vi "Begin.vi"(8 "error in":errorcluster) -> (0 "error out":T1)   [LabVIEW 2014]
doc: "Called before other user functions, this VI is expected to open initial I/O refnums, load in file data, and do all program initialization. Notice that the <B>error out</B> terminal is simply used for data flow. Wiring it to other structures or subVIs ensures that this VI runs first."
uses:
  ErrorOut.ctl
  <vilib>/Rock Robotics/WPI/SafetyOutput/WPI_SafetyOutputConfigMenu.ctl
  <vilib>/Rock Robotics/WPI/DriverStation/WPI_DriverStationRobotMode2.ctl
  <vilib>/Rock Robotics/WPI/Joystick/WPI_JoystickDeviceEnum.ctl
  <vilib>/Rock Robotics/SystemInterfaces/AI/FPGA_AIGyroChannel.ctl
  Robot Global Data.vi
  <vilib>/Rock Robotics/Network Tables/SD Write String Array.vi
  <vilib>/Rock Robotics/WPI/RobotDrive/WPI_RobotDriveOpen4MotorWithCANTalonSRX.vi
  <vilib>/Rock Robotics/WPI/MotorControl/WPI_MotorControlOpenCANTalonSRX.vi
  <vilib>/Rock Robotics/WPI/Compressor/WPI_CompressorGetSetRefNum.vi
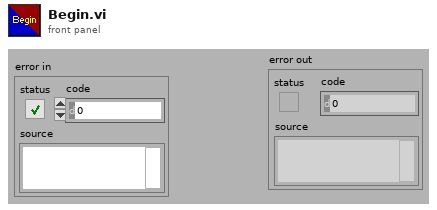
[diagram p1: front panel]
types:
  T1 = typedef "ErrorOut.ctl" = errorcluster
  T2 = typedef "FPGA_AIGyroChannel.ctl" = enum8{"AI 0", "AI 1", "Invalid"}
  T3 = typedef "WPI_JoystickDeviceEnum.ctl" = enum16{"USB 0", "USB 1", "USB 2", "USB 3", "USB 4", "USB 5"}
  T4 = typedef "WPI_DriverStationRobotMode2.ctl" = enum16{"Autonomous Disabled", "Autonomous Enabled", "Teleop Disabled", "Teleop Enabled", "Disconnected", "Finish", "Test Disabled", "Test Enabled", "Emergency Stopped"}
  T5 = typedef "WPI_SafetyOutputConfigMenu.ctl" = enum16{"Enable", "Disable"}
  T6 = typedef "WPI_JoystickDevRef.ctl" = cluster{"Device":T3}
  T7 = typedef "WPI_RobotDriveDevRef.ctl" = cluster{"DevStatus":errorcluster, "Motors[]":T8[], "Square Inputs":bool, "Max Output":dbl}
  T8 = typedef "WPI_MotorControlDeviceRef.ctl" = cluster{"DeviceStatus":errorcluster, "Type":T9, "PWM":cluster{"Controller":T10, "PWM Channel":T11, "DeadBand":T12}, "CAN":cluster{"Device Number":u8, "Control Mode":T13, "Semaphore":T14, "Max Vout":dbl, "TalonSRX Control Mode":T15}, "Invert":bool, "TransformRef":T16, "InvTransformRef":T16}
  T9 = typedef "WPI_MotorControlType.ctl" = enum16{"PWM", "CAN", "CANTalonSRX"}
  T10 = typedef "FPGA_TypedefDigitalModule.ctl" = enum16{"Controller 1"}
  T11 = typedef "FPGA_DIOPWMChannel.ctl" = enum8{"PWM 0", "PWM 1", "PWM 2", "PWM 3", "PWM 4", "PWM 5", "PWM 6", "PWM 7", "PWM 8", "PWM 9", "PWM MXP 0", "PWM MXP 1", "PWM MXP 2", "PWM MXP 3", "PWM MXP 4", "PWM MXP 5", "PWM MXP 6", "PWM MXP 7", "PWM MXP 8", "PWM MXP 9", "Invalid"}
  T12 = typedef "WPI_PWMDeadband.ctl" = cluster{"Name":string, "maxPositivePwm":i32, "minPositivePwm":i32, "centerPwm":i32, "maxNegativePwm":i32, "minNegativePwm":i32, "angularRange":u16}
  T13 = typedef "WPI_CANJaguar_ControlMode.ctl" = enum8{"Percent VBus", "Current", "Speed", "Position", "Voltage"}
  T14 = typedef "Semaphore RefNum" = refnum<k1>
  T15 = typedef "WPI_CANTalonSRX_APIControlMode.ctl" = enum8{"Percent VBus", "Speed", "Position", "Slave", "Unchanged / Invalid"}
  T16 = typedef "WPI_PWMTransform_ConPane.ctl" = refnum<vi>
  T17 = typedef "WPI_CompressorDevRef.ctl" = cluster{"DevStatus":errorcluster, "Pneumatics Control Module":u8}
  T18 = typedef "WPI_GyroDevRef.ctl" = cluster{"DevStatus":errorcluster, "Analog Module":T19, "Analog Channel":T20, "Offset":dbl, "Gain (VoltsPerDegree/Second)":dbl}
  T19 = typedef "FPGA_TypedefAnalogModule.ctl" = enum16{"Controller 1"}
  T20 = typedef "FPGA_AIChannel.ctl" = enum8{"AI 0", "AI 1", "AI 2", "AI 3", "AI MXP 0", "AI MXP 1", "AI MXP 2", "AI MXP 3", "Invalid"}
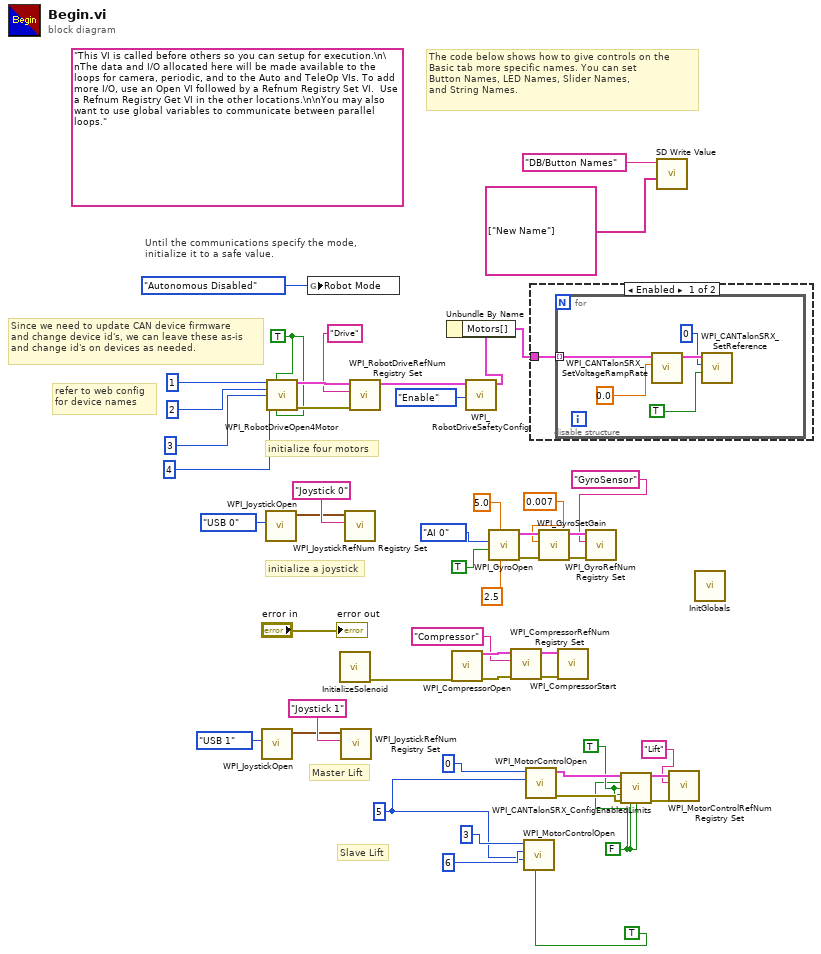
[diagram p0: block diagram]
diagram:
  w17 = FALSE
  w18 = TRUE
  w21 = 5
  w35 = TRUE
  (unwired) "This VI is called before others so you can setup for execution.\n\nThe data and I/O allocated here will be made available to the loops for camera, periodic, and to the Auto and TeleOp VIs. To add more I/O, use an Open VI followed by a Refnum Registry Set VI.  Use a Refnum Registry Get VI in the other locations.\n\nYou may also want to use global variables to communicate between parallel loops."
  # "Slave Lift"
  # "Master Lift"
  # "refer to web config\nfor device names"
  # "Since we need to update CAN device firmware\nand change device id's, we can leave these as-is\nand change id's on devices as needed."
  # "The code below shows how to give controls on the\nBasic tab more specific names. You can set\nButton Names, LED Names, Slider Names,\nand String Names."
  # "initialize a joystick"
  # "Until the communications specify the mode,\ninitialize it to a safe value."
  # "initialize four motors"
  n1 = call <vilib>:"WPI_JoystickOpen.vi"("JoystickDevice"=WPI_JoystickDeviceEnum."USB 1") -> ("JoystickDevRef"=w26:T6)  [unwired: 10 in]
  n2 = call <vilib>:"WPI_JoystickOpen.vi"("JoystickDevice"=WPI_JoystickDeviceEnum."USB 0") -> ("JoystickDevRef"=w43:T6)  [unwired: 10 in]
  n3 = call-poly <vilib>:"WPI_RobotDriveOpen4Motor.vi"("Rear Left Motor"=u8 1, "Rear Left Motor Inverted"=w35, "Rear Right Motor"=u8 2, "Front Left Motor"=u8 3, "Front Right Motor"=u8 4, "Front Left Motor Inverted"=w35) -> ("RobotDriveDevRef"=w50:T7, "error out"=w48:errorcluster)  [unwired: 8 in]
  n4 = global write "Robot Global Data.vi" "Robot Mode"(WPI_DriverStationRobotMode2."Autonomous Disabled" ("Robot Mode")) -> ()
  n5 = call "InitializeSolenoid.vi"() -> ("error out"=w28:T1)  [unwired: 11 in]
  n6 = call <vilib>:"WPI_JoystickRefNum Registry Set.vi"("refnum name"="Joystick 1", "JoystickDevRef"=w26) -> ()  [unwired: 8 in, 2 out]
  n7 = call <vilib>:"WPI_JoystickRefNum Registry Set.vi"("refnum name"="Joystick 0", "JoystickDevRef"=w43) -> ()  [unwired: 8 in, 2 out]
  n8 = call <vilib>:"WPI_RobotDriveRefNum Registry Set.vi"("error in (no error)"=w48, "refnum name"="Drive", "RobotDriveDevRef"=w50) -> ("RobotDriveDevRef"=w47:T7)  [unwired: 8 out]
  n9 = call <vilib>:"WPI_CompressorOpen.vi"("error in (no error)"=w28) -> ("CompressorDevRef"=w33:T17, "error out"=w34:errorcluster)  [unwired: 13 in]
  n10 = call <vilib>:"WPI_RobotDriveSafetyConfig.vi"("mode"=WPI_SafetyOutputConfigMenu."Enable", "RobotDriveDevRef"=w47) -> ("RobotDriveDevRef"=w12:T7)  [unwired: 8 in, 1 out]
  n11 = Unbundle By Name(w12) -> ("Motors[]"=w11:T8[])
  n12 = call <vilib>:"WPI_GyroOpen.vi"("Calibrated Center Voltage"=2.5, "Calibration Time (s)"=5.0, "Calibrate On Open"=TRUE, "Analog Channel"=FPGA_AIGyroChannel."AI 0") -> ("error out"=w8:errorcluster, "GyroDevRef"=w7:T18)  [unwired: 5 in, 1 out]
  n13 = call <vilib>:"WPI_CompressorRefNum Registry Set.vi"("error in (no error)"=w34, "refnum name"="Compressor", "CompressorDevRef"=w33) -> ("error out"=w31:errorcluster, "CompressorDevRef"=w30:T17)  [unwired: 7 in]
  n14 = call-poly <vilib>:"WPI_MotorControlOpen.vi"("Invert"=TRUE, "Master Device Number"=w21, "Device Number"=6, "Control Mode"=3) -> ()  [unwired: 6 in, 2 out]
  n15 = call-poly <vilib>:"WPI_MotorControlOpen.vi"("Device Number"=w21, "Control Mode"=0) -> ("error out"=w20:errorcluster, "MotorControlDeviceRef"=w19:T8)  [unwired: 8 in]
  n16 = disable-structure shown="Enabled" {
    disable-tunnel: w11 -> [w51 _]
    frame Enabled {
      n17 = for {
        tunnel: w51 -> [w55] mode=indexing
        n18 = call <vilib>:"WPI_CANTalonSRX_SetVoltageRampRate.vi"("Throttle Ramp Rate (percent/s)"=0.0, "CAN Talon SRX Ref"=w55) -> ("CAN Talon SRX Ref Out"=w54:T8)  [unwired: 8 in, 1 out]
        n19 = call <vilib>:"WPI_CANTalonSRX_SetReference.vi"("Reverse Feedback Sensor"=TRUE, "Feedback Reference"=0, "CAN Talon SRX Ref"=w54) -> ()  [unwired: 7 in, 2 out]
      }
    }
    frame Disabled {
    }
  }
  n20 = call <vilib>:"WPI_GyroSetGain.vi"("error in (no error)"=w8, "Gain (VoltsPerDegree/Second)"=0.007, "GyroDevRef"=w7) -> ("error out"=w5:errorcluster, "GyroDevRef"=w4:T18)  [unwired: 7 in]
  n21 = call <vilib>:"WPI_CompressorStart.vi"("error in (no error)"=w31, "CompressorDevRef"=w30) -> ()  [unwired: 8 in, 2 out]
  n22 = call <vilib>:"WPI_GyroRefNum Registry Set.vi"("error in (no error)"=w5, "refnum name"="GyroSensor", "GyroDevRef"=w4) -> ()  [unwired: 7 in, 2 out]
  n23 = call <vilib>:"WPI_CANTalonSRX_ConfigEnabledLimits.vi"("CAN Talon SRX Ref"=w19, "Override Limit Switches"=w17, "Forward Limit Switch Enable"=w18, "Reverse Limit Switch Enable"=w18, "error in (no error)"=w20, "Forward Soft Limit Enable"=w17, "Reverse Soft Limit Enable"=w17) -> ("CAN Talon SRX Ref Out"=w15:T8, "error out"=w16:errorcluster)  [unwired: 7 in]
  n24 = call-poly <vilib>:"SD Write Value.vi"("String Array"=string[] ["New Name"], "Name"="DB/Button Names") -> ()  [unwired: 8 in, 2 out]
  n25 = call <vilib>:"WPI_MotorControlRefNum Registry Set.vi"("error in (no error)"=w16, "refnum name"="Lift", "MotorControlDevRef"=w15) -> ()  [unwired: 7 in, 2 out]
  n26 = call "InitGlobals.vi"() -> ()  [unwired: 12 in]
  "error out" <- "error in"
